vi "AddReader.vi"(8 "error in (no error)":errorcluster, 10 "Reader to add":refnum<class "BaseReader.lvclass">, 11 "MultiReader in":refnum<class "MultiReader.lvclass">) -> (0 "error out":errorcluster, 3 "MultiReader out":refnum<class "MultiReader.lvclass">)   [LabVIEW 2013, in "MultiReader.lvclass"]
doc: "Adds a sub-reader to the multi reader. When sending/reading, all operations done on the multireader will be done on all the sub-readers it contains"
uses:
  MultiReader.lvclass
  BaseReader/BaseReader.lvclass
  MultiReader.lvclass/MultiReader.ctl
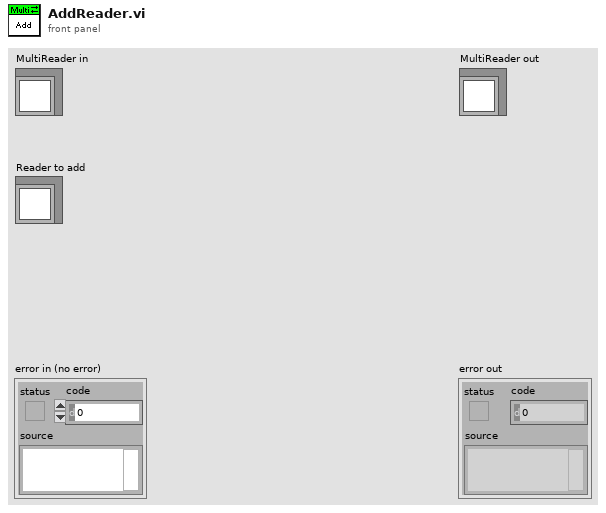
[diagram p1: front panel]
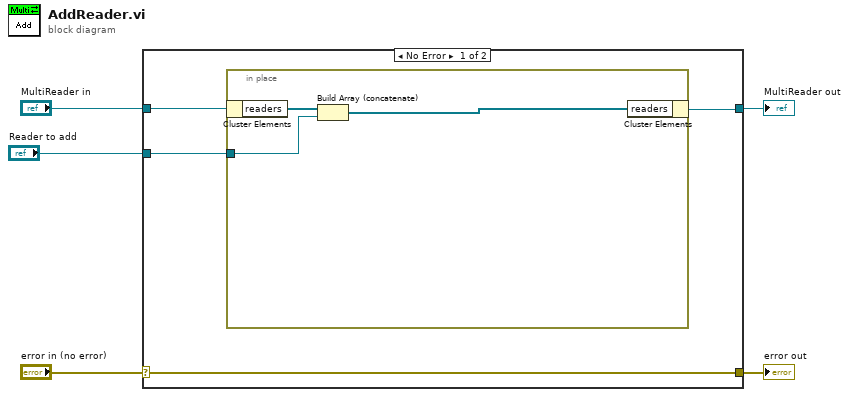
[diagram p0: block diagram]
diagram:
  n1 = case shown="No Error" "error in (no error)" {
    selector: "error in (no error)" -> [w9 w14]
    tunnel: [w9 w14] -> w4
    tunnel: [w6 w13] -> w2
    tunnel: "MultiReader in" -> [w8 w13]
    tunnel: "Reader to add" -> [w7 _]
    frame No Error {
      n2 = in-place {
        in-place-border: w7 -> [w11]
        n3 = in-place-cluster #1(w8) -> ("readers"=w12:refnum<class "BaseReader.lvclass">[])
        n4 = Build Array (concatenate)(w12, w11) -> (w10:refnum<class "BaseReader.lvclass">[])
        n5 = in-place-cluster #1("readers"=w10) -> (w6:refnum<class "MultiReader.lvclass">)
      }
    }
    frame Error {
    }
  }
  "error out" <- w4
  "MultiReader out" <- w2
